vi "XY Graph Get Plot Name & Scale Arrays.vi"(8 "error in":errorcluster, 10 "Scale Labels in":string[](array[string]), 11 "Plot Names in":string[](array[string])) -> (0 "error out":errorcluster, 1 "Alternating Axes?":bool, 2 "Plot Scales Array":T1(array[cluster]), 3 "Plot Names Array":string[](array[string]))   [LabVIEW 2021, in "XY Graph Add-Ons.lvlib"]
uses:
  XY Graph Add-Ons.lvlib
  <vilib>/Utility/error.llb/Error Cluster From Error Code.vi
  <vilib>/ErrorRing/Error Ring.xnode
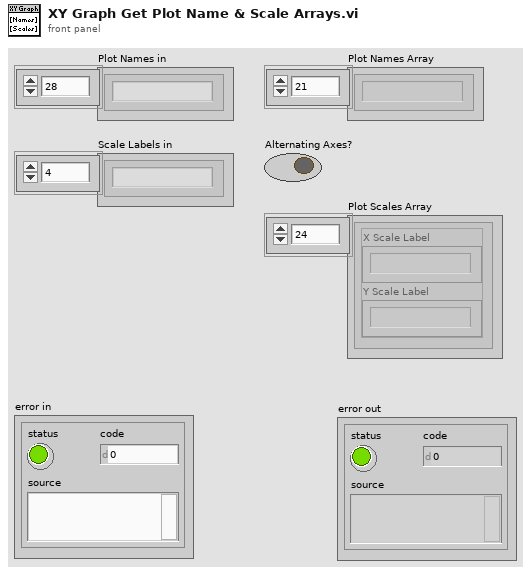
[diagram p1: front panel]
types:
  T1 = cluster{"X Scale Label":string, "Y Scale Label":string}[]
  T2 = cluster{"Scale Label":string, "Scale Label":string}
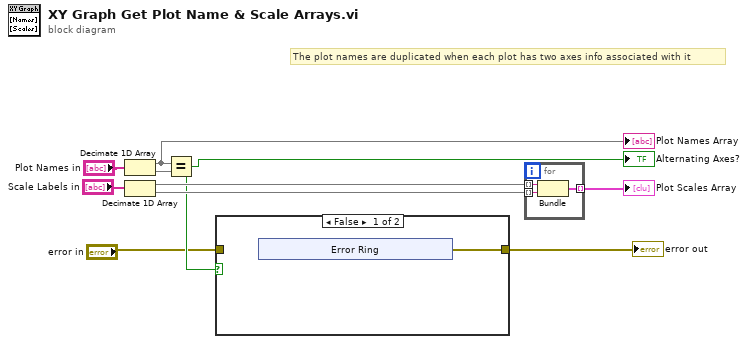
[diagram p0: block diagram]
diagram:
  # "The plot names are duplicated when each plot has two axes info associated with it"
  n1 = Decimate 1D Array("Plot Names in") -> (w6:string[], w5:string[])
  "Plot Names Array" <- w6
  n2 = Decimate 1D Array("Scale Labels in") -> (w8:string[], w9:string[])
  n3 = Equal?(x=w6, y=w5) -> (x = y?=w3:bool)
  "Alternating Axes?" <- w3
  n4 = case shown="False" w3 {
    tunnel: [w11 w16] -> w2
    tunnel: "error in" -> [_ w16]
    frame False {
      n5 = xnode "Error Ring"() -> ("error out"=w11:errorcluster)
    }
    frame True {
    }
  }
  "error out" <- w2
  n6 = for {
    tunnel: w8 -> [w19] mode=indexing
    tunnel: w9 -> [w18] mode=indexing
    tunnel: [w17] -> w10 mode=indexing
    n7 = Bundle("Scale Label"=w19, "Scale Label"=w18) -> (w17:T2)  [unwired: 1 in]
  }
  "Plot Scales Array" <- w10
